vi "ST5 Write Param.vi"(0 "Port COM":refnum<visa-resource-name>, 1 "Vitesse":dbl=0.08399999999999999 min=0.0042 max=133.3333 step=0.0042 format="%#.4g", 2 "Accél":dbl=0.167 caption="Accélération (Tour/s/s)" min=0.167 max=5461.167 step=0.167 format="%#.3g", 5 "Parameters":u16(ring) items=["Velocity", "Acceleration", "Deceleration", "Max Acceleration", "Zero", "Save", "Encoder Res", "Clear Alarm", "Home Search", "Motor Enable", "Motor Disable", "Out1", "Out2", "Out3", "Out4"], 7 "Décél":dbl=0.167 caption="Décélération (Tour/s/s)" min=0.167 max=5461.167 step=0.167 format="%#.3g", 9 "Accél Max":dbl=0.167 caption="Accélération Max (Tour/s/s)" min=0.167 max=5461.167 step=0.167 format="%#.3g", 11 "error in (no error)":errorcluster, 12 "Microstep Res(Pas/Tour)":dbl=200.0 min=200.0 max=51200.0 step=1.0, 13 "HomeInput":u8=1 caption="Home Input" min=1 max=8 step=1, 14 "Output Active":bool) -> (4 "Port COM Out":refnum<visa-resource-name>, 15 "error out":errorcluster)   [LabVIEW 2019]
doc: "Ce Vi envoie les chaînes de commande au contrôlleur de moteur ST5-Q et vérifie si une réponse se trouve dans le buffer du port série"
uses:
  <userlib>/ST5/StatesConst.ctl
panel:
  out "Réponse":string
  out "Commande":string
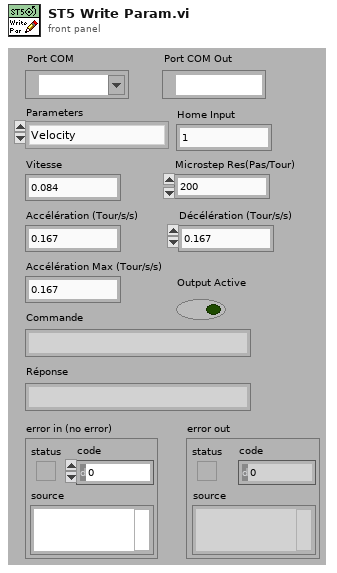
[diagram p1: front panel]
types:
  T1 = typedef "StatesConst.ctl" = enum16{"SendCom", "Read", "End"}
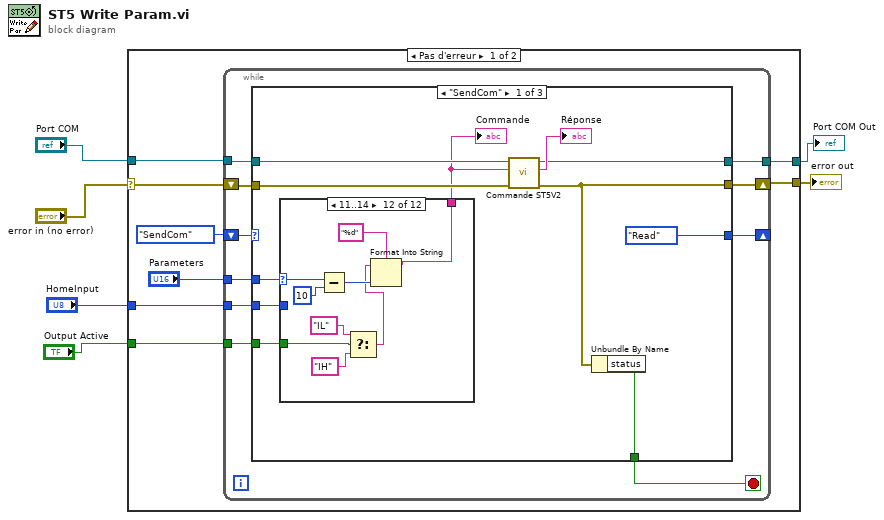
[diagram p0: block diagram]
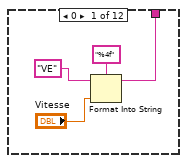
[diagram p2: hidden frame]
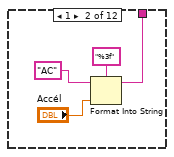
[diagram p3: hidden frame]
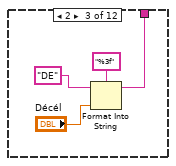
[diagram p4: hidden frame]
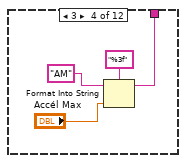
[diagram p5: hidden frame]
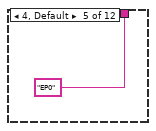
[diagram p6: hidden frame]
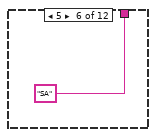
[diagram p7: hidden frame]
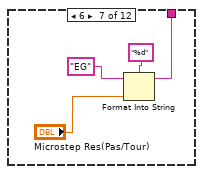
[diagram p8: hidden frame]
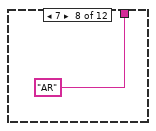
[diagram p9: hidden frame]
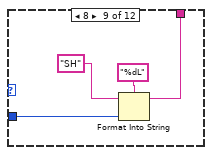
[diagram p10: hidden frame]
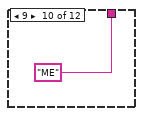
[diagram p11: hidden frame]
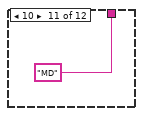
[diagram p12: hidden frame]
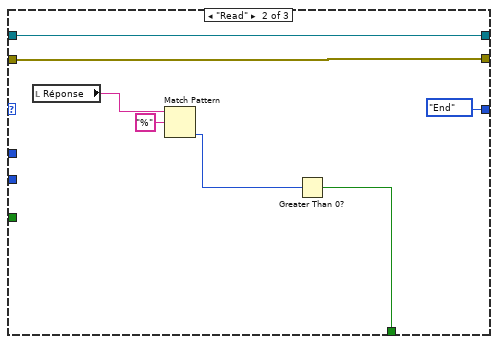
[diagram p13: hidden frame]
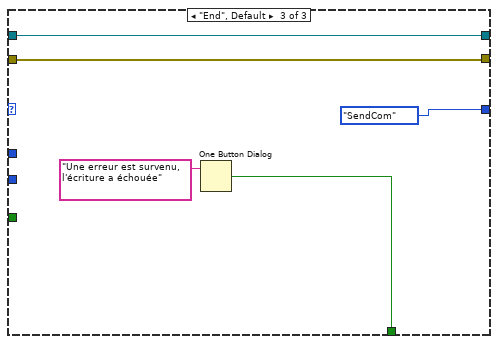
[diagram p14: hidden frame]
diagram:
  n1 = case shown="Pas d'erreur" "error in (no error)" {
    selector: "error in (no error)" -> [w13 w87]
    tunnel: "Port COM" -> [w14 w86]
    tunnel: [w11 w87] -> w4
    tunnel: [w9 w86] -> w3
    tunnel: "HomeInput" -> [w8 _]
    tunnel: "Output Active" -> [w7 _]
    frame No Error {
      n2 = while {
        tunnel: w14 -> [w24]
        shift-right: [w21] -> w11
        shift-left: w13 -> [w23]
        shift-right: [w20] -> _
        shift-left: StatesConst."SendCom" ("Énum") -> [w22]
        tunnel: "Parameters" -> [w19]
        tunnel: [w17] -> w9
        tunnel: w8 -> [w16]
        tunnel: w7 -> [w15]
        stop <- w18 stop-if-true
        n3 = case shown="\"SendCom\"" w22 {
          tunnel: w24 -> [w33 w74 w81]
          tunnel: w23 -> [w32 w79 w84]
          tunnel: [w31 w79 w84] -> w21
          tunnel: [StatesConst."Read" ("Énum") StatesConst."End" ("Énum") StatesConst."SendCom" ("Énum")] -> w20
          tunnel: w19 -> [w29 _ _]
          tunnel: [w35 w75 w82] -> w18
          tunnel: [w27 w74 w81] -> w17
          tunnel: w16 -> [w26 _ _]
          tunnel: w15 -> [w25 _ _]
          frame "SendCom" {
            n4 = case shown="11..14" w29 {
              selector: w29 -> [_ _ _ _ _ _ _ _ _ _ _ w73]
              tunnel: [w36 w40 w44 w48 "EP0" "SA" w55 "AR" w60 "ME" "MD" w65] -> w28
              tunnel: w26 -> [_ _ _ _ _ _ _ _ w59 _ _ _]
              tunnel: w25 -> [_ _ _ _ _ _ _ _ _ _ _ w72]
              frame 0 {
                n5 = Format Into String(format string="%4f" ("chaîne de format"), initial string="VE", "Vitesse") -> (resulting string=w36:string)  [unwired: 1 in, 1 out]
              }
              frame 1 {
                n6 = Format Into String(format string="%3f" ("chaîne de format"), initial string="AC", "Accél") -> (resulting string=w40:string)  [unwired: 1 in, 1 out]
              }
              frame 2 {
                n7 = Format Into String(format string="%3f" ("chaîne de format"), initial string="DE", "Décél") -> (resulting string=w44:string)  [unwired: 1 in, 1 out]
              }
              frame 3 {
                n8 = Format Into String(format string="%3f" ("chaîne de format"), initial string="AM", "Accél Max") -> (resulting string=w48:string)  [unwired: 1 in, 1 out]
              }
              frame 4, Default {
              }
              frame 5 {
              }
              frame 6 {
                n9 = Format Into String(format string="%d" ("chaîne de format"), initial string="EG", "Microstep Res(Pas/Tour)") -> (resulting string=w55:string)  [unwired: 1 in, 1 out]
              }
              frame 7 {
              }
              frame 8 {
                n10 = Format Into String(format string="%dL" ("chaîne de format"), initial string="SH", w59) -> (resulting string=w60:string)  [unwired: 1 in, 1 out]
              }
              frame 9 {
              }
              frame 10 {
              }
              frame 11..14 {
                n11 = Subtract(x=w73, y=u16 10) -> (x-y=w69:u16)
                n12 = Select(t="IL", s=w72, f="IH") -> (s? t:f=w67:string)
                n13 = Format Into String(format string="%d" ("chaîne de format"), initial string=w67, w69) -> (resulting string=w65:string)  [unwired: 1 in, 1 out]
              }
            }
            "Commande" <- w28
            n14 = call <userlib>:"Commande ST5V2.vi"("error in (no error)"=w32, "Commande"=w28, "Port COM"=w33) -> ("error out"=w31:errorcluster, "Réponse"=→"Réponse":string, "Port Out"=w27:refnum<visa-resource-name>)  [unwired: 1 in, 1 out]
            n15 = Unbundle By Name(w31) -> ("status"=w35:bool)
          }
          frame "Read" {
            n16 = local read "Réponse"() -> (w78:string)
            n17 = Match Pattern(string=w78, regular expression="%" ("expression régulière")) -> (offset past match=w76:i32)  [unwired: 1 in, 3 out]
            n18 = Greater Than 0?(x=w76) -> (x > 0?=w75:bool)
          }
          frame "End", Default {
            n19 = One Button Dialog(message="Une erreur est survenu, l'écriture a échouée") -> (true=w82:bool)  [unwired: 1 in]
          }
        }
      }
    }
    frame Error {
    }
  }
  "error out" <- w4
  "Port COM Out" <- w3
